vi "WorkorderHandler_referenceProbe.vi"(1 "reference":T2) -> (0 "Boolean":bool)   [LabVIEW 2011]
doc: "Use this custom probe to probe a dqGOOP reference and view statistics and the data associated with the dqGOOP object. Additional conditions can be created that are useful for your particular class. Be sure to move or copy this VI to the user.lib\\_probes or the Default Data\\Probes directories."
uses:
  Software/DataStructures/WorkorderHandler_ObjectReference.ctl
  Software/DataStructures/WorkorderHandler_ObjectData.ctl
panel:
  in  "Tab Control":enum32{"reference", "condition"}(tab)
  out "pending":i32
  out "object state":u16(ring) items=["unlocked", "locked", "not a reference"]
  out "object name":string
  out "reference":u32 format="%08x"
  out "data":T1
  in  "object state 2":u16(ring) items=["unlocked", "locked", "not a reference"]
  in  "object sate is:":bool
  # "Pause if any of the following:"
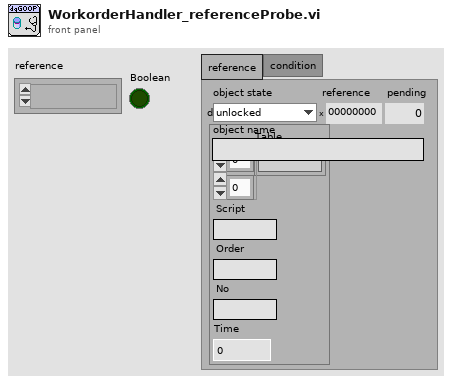
[diagram p1: front panel]
types:
  T1 = typedef "WorkorderHandler_ObjectData.ctl" = cluster{"Table":string[][], "Script":string, "Order":string, "No":string, "Time":dbl}
  T2 = typedef "WorkorderHandler_ObjectReference.ctl" = refnum<k1>
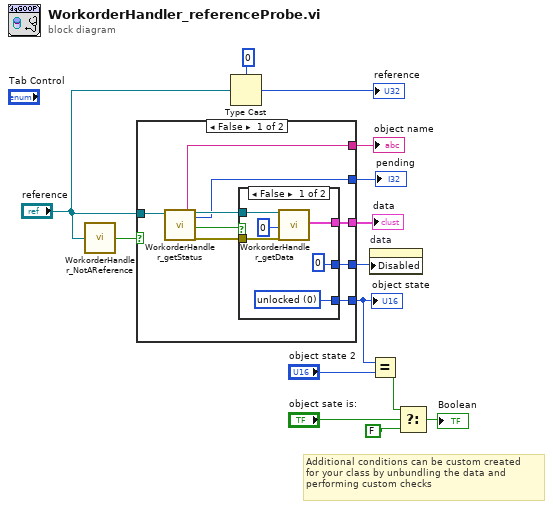
[diagram p0: block diagram]
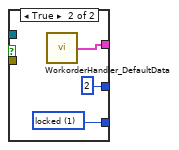
[diagram p2: hidden frame]
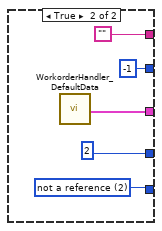
[diagram p3: hidden frame]
diagram:
  # "Additional conditions can be custom created\nfor your class by unbundling the data and\nperforming custom checks"
  n1 = call "WorkorderHandler_NotAReference.vi"("reference"="reference") -> ("not a reference?"=w6:bool)
  n2 = case shown="False" w6 {
    tunnel: [w21 w36] -> w14
    tunnel: [w20 u8 2 ("Disabled")] -> w13
    tunnel: [w19 ""] -> w12
    tunnel: [w16 w34] -> w5
    tunnel: "reference" -> [w18 _]
    tunnel: [w15 -1 ("methods pending lock")] -> w1
    frame False {
      n3 = call "WorkorderHandler_getStatus.vi"("reference"=w18) -> ("object name"=w19:string, "duplicate reference"=w23:T2, "methods pending lock"=w15:i32, "object locked"=w17:bool, "error out"=w22:errorcluster)  [unwired: 1 in, 13 out]
      n4 = case shown="False" w17 {
        tunnel: w23 -> [w29 _]
        tunnel: w22 -> [w28 _]
        tunnel: [w26 w32] -> w21
        tunnel: [u8 0 ("Disabled") u8 2 ("Disabled")] -> w20
        tunnel: [w24 w30] -> w16
        frame False {
          w24 = u16 0 items=["unlocked", "locked", "not a reference"] ("object state")
          n5 = call "WorkorderHandler_getData.vi"("reference"=w29, "timeout in ms (-1)"=0, "error in (no error)"=w28) -> ("data"=w26:T1)  [unwired: 16 out]
        }
        frame True {
          w30 = u16 1 items=["unlocked", "locked", "not a reference"] ("object state")
          n6 = call "WorkorderHandler_DefaultData.vi"() -> ("data"=w32:T1)
        }
      }
    }
    frame True {
      w34 = u16 2 items=["unlocked", "locked", "not a reference"] ("object state")
      n7 = call "WorkorderHandler_DefaultData.vi"() -> ("data"=w36:T1)
    }
  }
  "data" <- w14
  "object name" <- w12
  "object state" <- w5
  "pending" <- w1
  n8 = Type Cast(type=u32 0 ("Reference"), x="reference") -> (*(type *) &x=→"reference":u32)
  n9 = property on="data" class="Clust (strict)"("Disabled"=w13) -> ()  [unwired: 2 in, 2 out]
  n10 = Equal?(x=w5, y="object state 2") -> (x = y?=w3:bool)
  n11 = Select(t=w3, s="object sate is:", f=FALSE) -> (s? t:f=→"Boolean":bool)
